vi "ArmLimit.vi"(9 "Extend":dbl, 10 "Lift":dbl) -> (1 "Extend":dbl, 2 "Lift":dbl)   [LabVIEW 2020]
uses:
  GeneralPurpose/3Dpoint.ctl
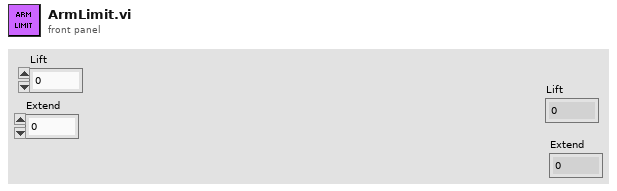
[diagram p1: front panel]
types:
  T1 = typedef "3Dpoint.ctl" = cluster{"X":dbl, "Y":dbl, "Z":dbl}
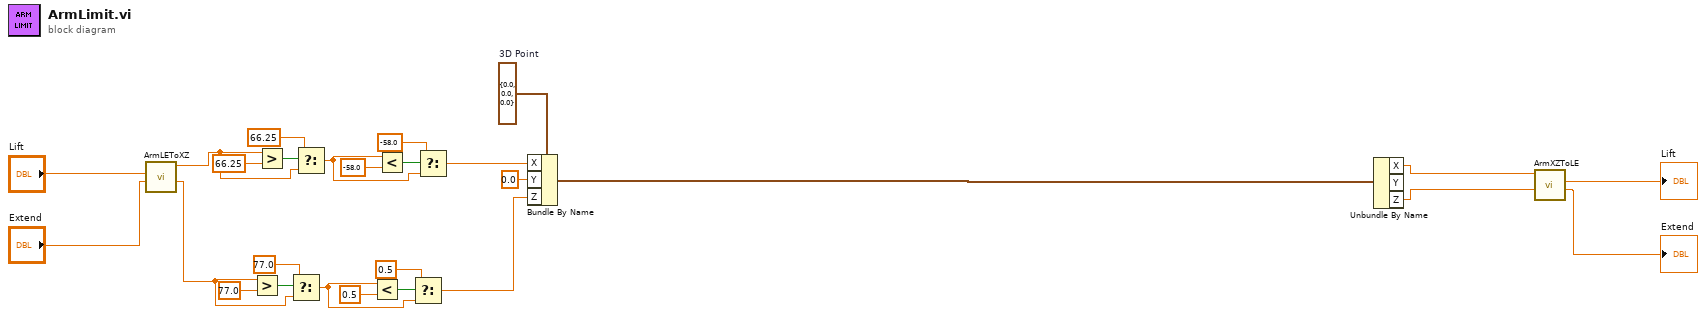
[diagram p0: block diagram]
diagram:
  w23 = T1 {"X"=0.0, "Y"=0.0, "Z"=0.0}  # 3D Point
  n1 = call "ArmLEToXZ.vi"("Extend"="Extend", "Lift"="Lift") -> ("z"=w3:dbl, "x"=w14:dbl)  [unwired: 8 in]
  n2 = Greater?(x=w3, y=77.0) -> (0:w11:bool)
  n3 = Greater?(x=w14, y=66.25) -> (0:w20:bool)
  n4 = Select(t=77.0, s=w11, f=w3) -> (s? t:f=w6:dbl)
  n5 = Select(t=66.25, s=w20, f=w14) -> (s? t:f=w15:dbl)
  n6 = Less?(x=w6, y=0.5) -> (x < y?=w10:bool)
  n7 = Less?(x=w15, y=-58.0) -> (x < y?=w19:bool)
  n8 = Select(t=0.5, s=w10, f=w6) -> (s? t:f=w4:dbl)
  n9 = Select(t=-58.0, s=w19, f=w15) -> (s? t:f=w12:dbl)
  n10 = Bundle By Name(cluster=w23, "X"=w12, "Y"=0.0, "Z"=w4) -> (w2:T1)
  n11 = Unbundle By Name(w2) -> ("X"=w22:dbl, "Z"=w21:dbl)  [unwired: 1 out]
  n12 = call "ArmXZToLE.vi"("Z"=w21, "X"=w22) -> ("Extend"=→"Extend":dbl, "Lift"=→"Lift":dbl)  [unwired: 8 in]
